vi "Constructor Testing.vi"() -> ()   [LabVIEW 2014]
uses:
  C:/Robotic Systems/Products/Surveyor/Software/Ground Station/Data/Mapping DLL/GMap.NET.Core.dll
  Data/Mapping DLL/GMap.NET.Core.dll
panel:
  out "Mode":i32(ring) items=["ServerOnly", "ServerAndCache", "CacheOnly"]
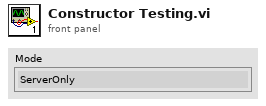
[diagram p1: front panel]
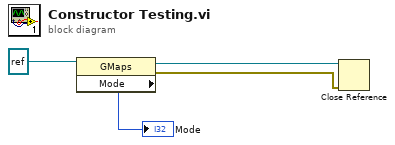
[diagram p0: block diagram]
diagram:
  n1 = property class="GMaps"(reference=refnum<k24> refnum) -> (reference out=w4:refnum<k24>, error out=w3:errorcluster, "Mode"=→"Mode":i32)  [unwired: 1 in]
  n2 = Close Reference(reference=w4, error in (no error)=w3) -> ()  [unwired: 1 out]
